vi "gauss.vi"() -> ()   [LabVIEW 2018]
uses:
  Control 1.ctl
  <vilib>/Analysis/4window.llb/windowTd.ctl
  <vilib>/DAQmx/write.llb/DAQmx Write (Analog 1D Wfm NChan NSamp).vi
  <vilib>/Analysis/1siggen.llb/General Gauss-Mod Sine.vi
  <vilib>/measure/maspectr.llb/FFT Power Spectrum and PSD for 1 Chan.vi
  <vilib>/DAQmx/create/channels.llb/DAQmx Create Channel (AO-Voltage-Basic).vi
  <vilib>/DAQmx/configure/timing.llb/DAQmx Timing (Sample Clock).vi
  <vilib>/DAQmx/miscellaneous.llb/DAQmx Fill In Error Info.vi
  <vilib>/Analysis/NI_AALBase.lvlib
  <vilib>/measure/NI_MAPro.lvlib
  <resource>/objmgr/daqmx.rc
  <vilib>/measure/NI_MABase.lvlib
  <vilib>/Analysis/NI_AALPro.lvlib
panel:
  in  "amplitude":dbl=1.0
  in  "delay":dbl
  in  "width":dbl=0.5
  out "Sampling rate":dbl=799999.9999999999
  in  "f2":dbl=300.0 format="%0.2f"
  in  "f1":dbl=100.0 format="%0.2f"
  in  "Test device":bool
  in  "Exit":bool
  out "Actual Sample Rate 2":dbl=800000.0 format="%0.2f"
  in  "Physical Channel(s)":tag="Dev3/ao0:1"
  in  "Min Voltage 2":dbl=-10.0
  in  "Max Voltage 2":dbl=10.0
  in  "Sample Clock Source":tag="OnboardClock"
  in  "Sample Rate 2":dbl=800000.0 format="%#_6p"
  in  "Pulser Cycles":i32=10
  out "Sample per Channel AO":dbl=26666.0
  in  "Pulse generator":T2={"Waveform Type"=2, "Amplitude"=1.0, "Frequency"=300.0} {"Frequency" format="%0.2p"; "Amplitude" format="%0.2p"; "Waveform Type" items=["Sine Wave", "Triangle Wave", "Square Wave", "Sawtooth Wave"]}
  in  "Duty cycle %":dbl=50.0 format="%#.2f"
  in  "samples 2":i32=300
  in  "Amplitude & Delay":cluster{"Amplitude":dbl, "Delay (s)":dbl}[](array[cluster])=[{"Amplitude"=5.0, "Delay (s)"=1.0}, {"Amplitude"=3.0, "Delay (s)"=8.0}, {"Amplitude"=1.0, "Delay (s)"=15.0}]
  in  "interpolation method":i32(ring)=1 items=["nearest", "linear", "spline", "cubic Hermite"]
  out "Pulse Train":waveform(dbl)(graph)={"t0"=timestamp(0 s since 1904-01-01), "dt"=1.25e-06, "Y"=[]}
  out "Waveform Graph 2":cluster{"f0":dbl, "df":dbl, "magnitude":dbl[]}[](graph)=[{"f0"=0.0, "df"=20.0, "magnitude"=array[20000 elements]}, {"f0"=0.0, "df"=20.0, "magnitude"=array[20000 elements]}, {"f0"=0.0, "df"=20.0, "magnitude"=array[20000 elements]}]
  in  "normalized bandwidth":dbl=0.5
  in  "attenuation (dB)":dbl=7.0
  out "Waveform Graph":waveform(dbl)[](graph)=[{"t0"=timestamp(0 s since 1904-01-01), "dt"=1.25e-06, "Y"=array[40000 elements]}, {"t0"=timestamp(0 s since 1904-01-01), "dt"=1.25e-06, "Y"=array[40000 elements]}, {"t0"=timestamp(0 s since 1904-01-01), "dt"=1.25e-06, "Y"=array[40000 elements]}]
  in  "center frequency (Hz)":dbl=200.0
  in  "delay (s)":dbl=0.025
  in  "delta t (s)":dbl=1.25e-06
  in  "samples":i32=40000
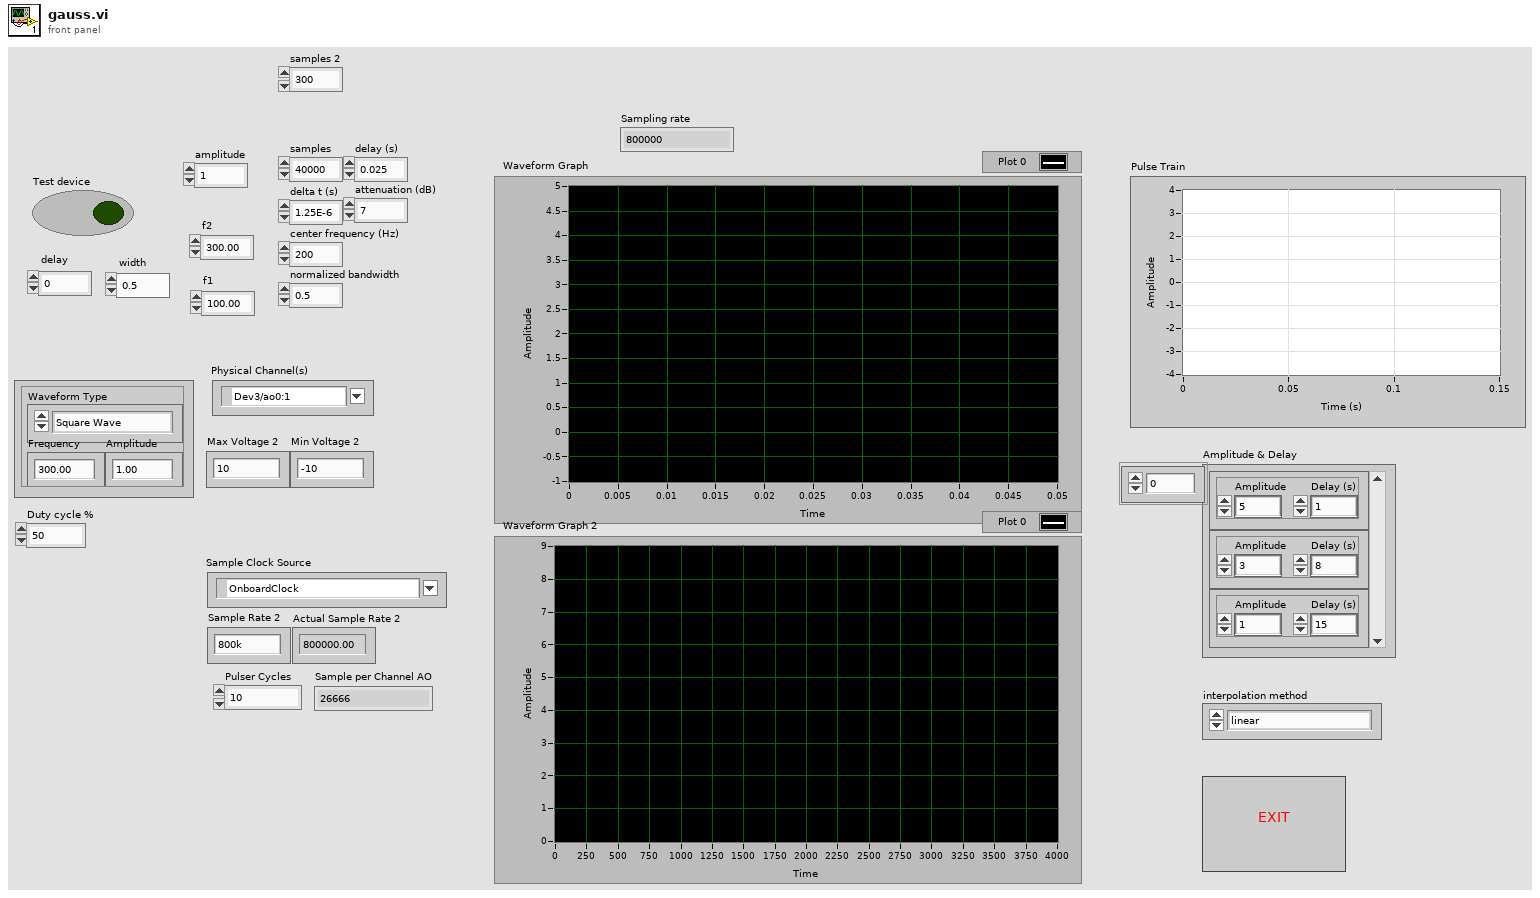
[diagram p1: front panel]
types:
  T1 = typedef "Control 1.ctl" = dbl
  T2 = cluster{"Waveform Type":u16, "Amplitude":T1, "Frequency":dbl}
  T3 = typedef "NI_AALPro.lvlib/windowTd.ctl" = u32
  T4 = enum16{"Sine Wave", "Triangle Wave", "Square Wave", "Sawtooth Wave"}
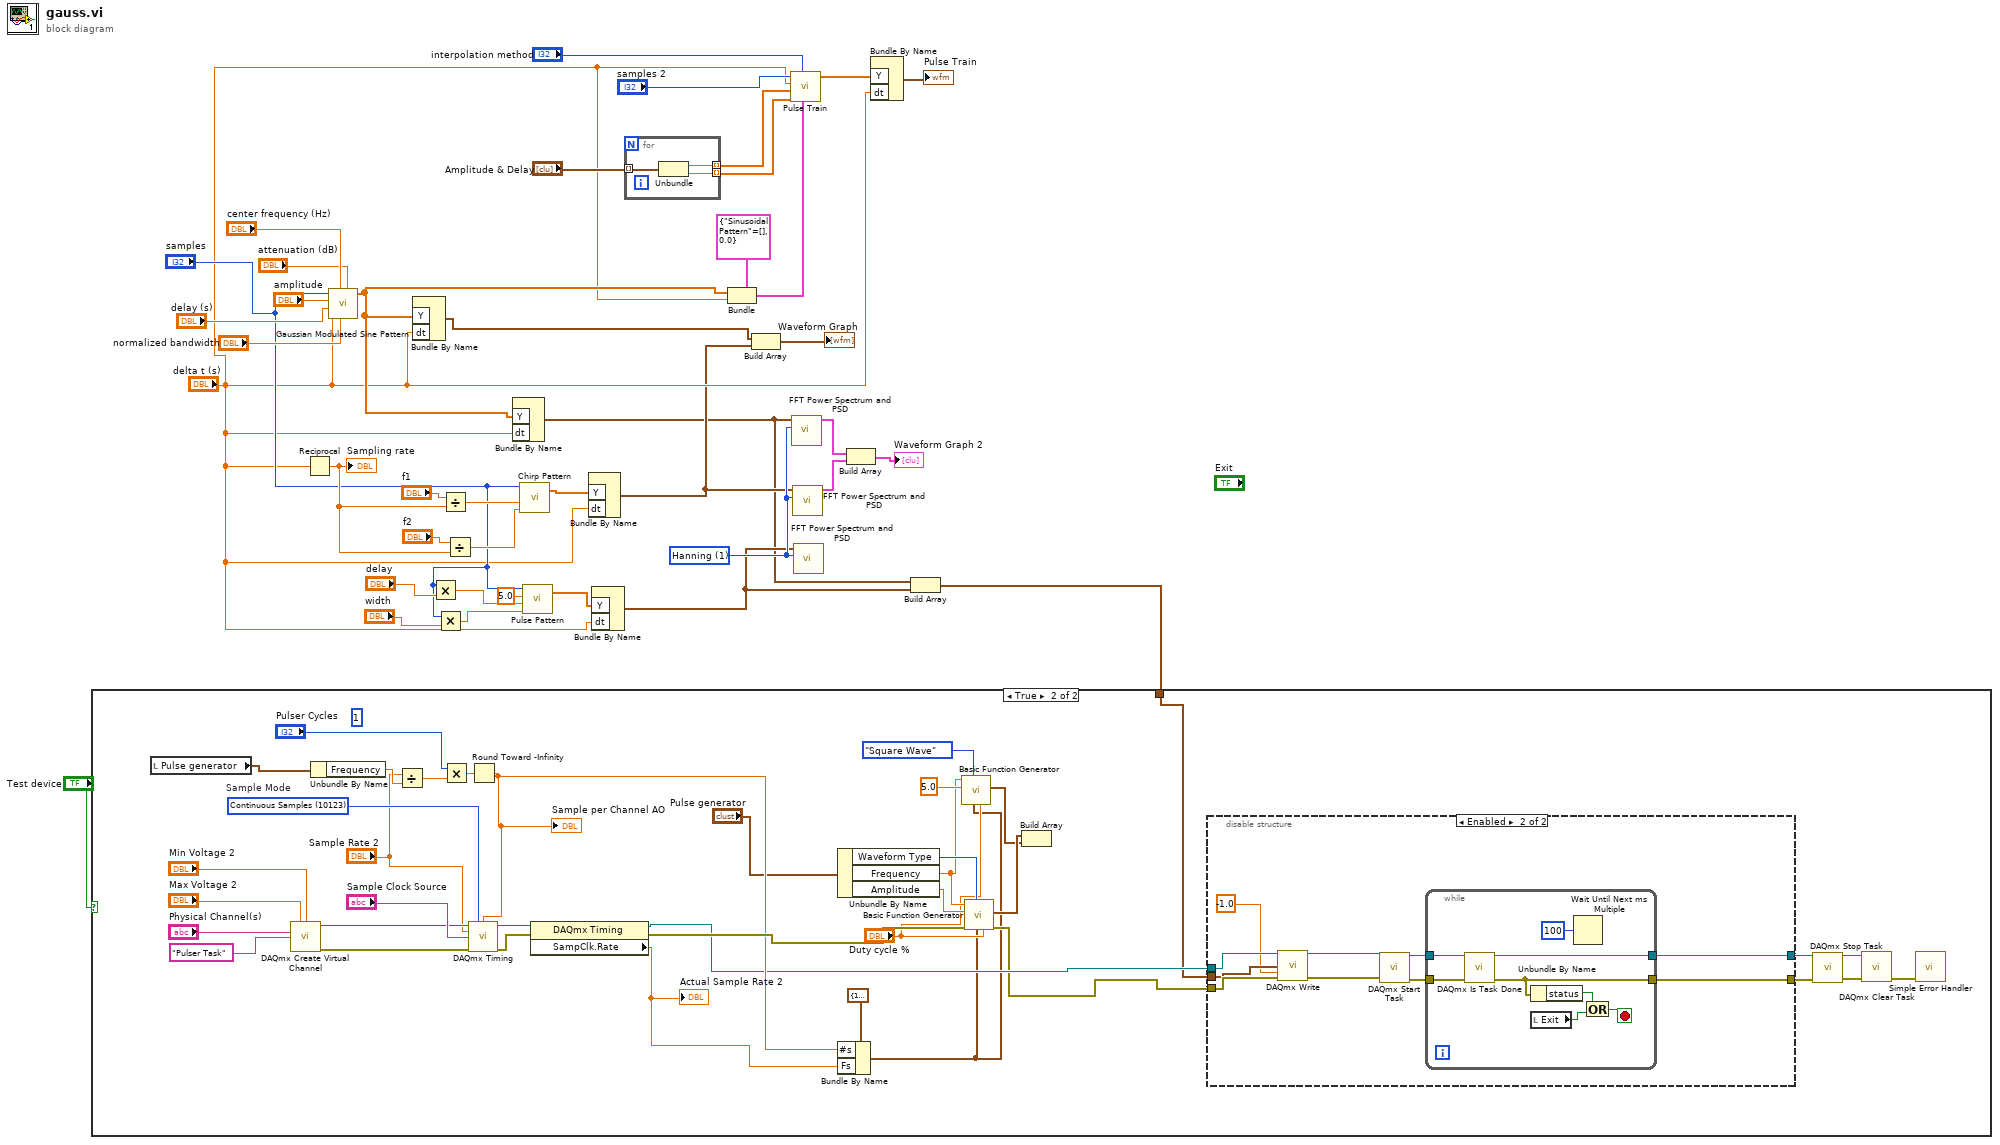
[diagram p0: block diagram]
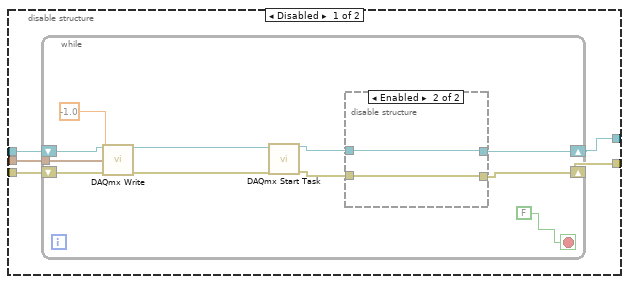
[diagram p3: hidden frame]
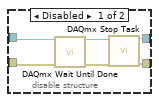
[diagram p4: hidden frame]
diagram:
  w8 = T3 1 items=["Rectangle"=0, "Hanning"=1, "Hamming"=2, "Blackman-Harris"=3, "Exact Blackman"=4, "Blackman"=5, "Flat Top"=6, "4 Term B-Harris "=7, "7 Term B-Harris"=8, "Low Sidelobe"=9, "Blackman Nuttall"=11, "Triangle"=30, "Bartlett-Hanning"=31, "Bohman"=32, "Parzen"=33, "Welch"=34, "Kaiser"=60, "Dolph-Chebyshev"=61, "Gaussian"=62] ("window")
  n1 = Reciprocal(x="delta t (s)") -> (1/x=w14:dbl)
  "Sampling rate" <- w14
  n2 = call <vilib>:"Gaussian Modulated Sine Pattern.vi"("attenuation (dB)"="attenuation (dB)", "normalized bandwidth"="normalized bandwidth", "center frequency (Hz)"="center frequency (Hz)", "delta t (s)"="delta t (s)", "delay (s)"="delay (s)", "amplitude"="amplitude", "samples"="samples") -> ("Gauss-Mod Sine Pattern"=w28:dbl[])  [unwired: 3 in, 1 out]
  n3 = Bundle By Name("Y"=w28, "dt"="delta t (s)") -> (w25:waveform(dbl))  [unwired: 1 in]
  n4 = Multiply(x="samples", y="delay") -> (x*y=w9:dbl)
  n5 = Multiply(x="samples", y="width") -> (x*y=w10:dbl)
  n6 = Divide(x="f1", y=w14) -> (x/y=w21:dbl)
  n7 = Divide(x="f2", y=w14) -> (x/y=w19:dbl)
  n8 = Bundle By Name("Y"=w28, "dt"="delta t (s)") -> (w1:waveform(dbl))  [unwired: 1 in]
  n9 = call <vilib>:"Chirp Pattern.vi"("f2"=w19, "f1"=w21, "samples"="samples") -> ("Chirp Pattern"=w23:dbl[])  [unwired: 1 in, 1 out]
  n10 = call <vilib>:"Pulse Pattern.vi"("width"=w10, "delay"=w9, "amplitude"=5.0, "samples"="samples") -> ("Pulse Pattern"=w15:dbl[])  [unwired: 1 out]
  n11 = Bundle By Name("Y"=w23, "dt"="delta t (s)") -> (w2:waveform(dbl))  [unwired: 1 in]
  n12 = Bundle By Name("Y"=w15, "dt"="delta t (s)") -> (w6:waveform(dbl))  [unwired: 1 in]
  n13 = for {
    tunnel: "Amplitude & Delay" -> [w43] mode=indexing
    tunnel: [w42] -> w32 mode=indexing
    tunnel: [w41] -> w31 mode=indexing
    n14 = Unbundle(w43) -> ("Amplitude"=w42:dbl, "Delay (s)"=w41:dbl)
  }
  n15 = Bundle(cluster=cluster{"Sinusoidal Pattern":dbl[], dbl} {"Sinusoidal Pattern"=[], 0.0} ("output cluster"), "Sinusoidal Pattern"=w28, "delta t (s)") -> (w27:cluster{"Sinusoidal Pattern":dbl[], dbl})
  n16 = Build Array(w25, w2) -> (→"Waveform Graph":waveform(dbl)[])
  n17 = call <vilib>:"Pulse Train.vi"("prototype spec"=w27, "interpolation method"="interpolation method", "Delay (s)"=w31, "Amplitude"=w32, "delta t of pulse train (s)"="delta t (s)", "samples"="samples 2") -> ("Pulse Train"=w35:dbl[])  [unwired: 4 in, 1 out]
  n18 = call-poly <vilib>:"FFT Power Spectrum and PSD.vi"("window"=w8, "time signal"=w1) -> ("Power Spectrum / PSD"=w17:cluster{"f0":dbl, "df":dbl, "magnitude":dbl[]})  [unwired: 6 in, 3 out]
  n19 = call-poly <vilib>:"FFT Power Spectrum and PSD.vi"("window"=w8, "time signal"=w2) -> ("Power Spectrum / PSD"=w18:cluster{"f0":dbl, "df":dbl, "magnitude":dbl[]})  [unwired: 6 in, 3 out]
  n20 = call-poly <vilib>:"FFT Power Spectrum and PSD.vi"("window"=w8, "time signal"=w6) -> ()  [unwired: 6 in, 4 out]
  n21 = Build Array(w17, w18) -> (→"Waveform Graph 2":cluster{"f0":dbl, "df":dbl, "magnitude":dbl[]}[])
  n22 = Bundle By Name("Y"=w35, "dt"="delta t (s)") -> (→"Pulse Train":waveform(dbl))  [unwired: 1 in]
  n23 = Build Array(w1, w6) -> (w5:waveform(dbl)[])
  n24 = case shown="True" "Test device" {
    tunnel: w5 -> [_ w44]
    frame False {
    }
    frame True {
      (unwired) 1 ("x")
      w79 = 10123 items=["Finite Samples"=10178, "Continuous Samples"=10123, "Hardware Timed Single Point"=12522]  # Sample Mode
      n25 = local read "Pulse generator"() -> (w63:T2)
      n26 = call-poly <vilib>:"DAQmx Create Virtual Channel.vi"("maximum value"="Max Voltage 2", "minimum value"="Min Voltage 2", "physical channels"="Physical Channel(s)", "name to assign"="Pulser Task") -> ("task out"=w70:refnum<k21>, "error out"=w69:errorcluster)  [unwired: 10 in]
      n27 = Unbundle By Name(w63) -> ("Frequency"=w68:dbl)
      n28 = Divide(x="Sample Rate 2", y=w68) -> (x/y=w66:dbl)
      n29 = Multiply(x="Pulser Cycles", y=w66) -> (x*y=w65:dbl)
      n30 = Round Toward -Infinity(1:w65) -> (0:w64:dbl)
      "Sample per Channel AO" <- w64
      n31 = call-poly <vilib>:"DAQmx Timing.vi"("task/channels in"=w70, "sample mode"=w79, "samples per channel"=w64, "rate"="Sample Rate 2", "source"="Sample Clock Source", "error in"=w69) -> ("task out"=w81:refnum<k21>, "error out"=w80:errorcluster)  [unwired: 8 in]
      n32 = property class="DAQmx Timing"(reference=w81, error in=w80) -> (reference out=w62:refnum<k21>, error out=w73:errorcluster, "SampClk.Rate"=w71:dbl)
      "Actual Sample Rate 2" <- w71
      n33 = Unbundle By Name("Pulse generator") -> ("Waveform Type"=w60:u16, "Frequency"=w56:dbl, "Amplitude"=w59:T1)
      n34 = Bundle By Name(cluster=cluster{"Fs":dbl, "#s":dbl} {"Fs"=1000.0, "#s"=1000.0} ("sampling info"), "#s"=w64, "Fs"=w71) -> (w51:cluster{"Fs":dbl, "#s":dbl})
      n35 = call <vilib>:"Basic Function Generator.vi"("square wave duty cycle (%)"="Duty cycle %", "sampling info"=w51, "signal type"=T4."Square Wave", "amplitude"=5.0, "frequency"=w56) -> ("signal out"=w52:waveform(dbl))  [unwired: 4 in, 2 out]
      n36 = call <vilib>:"Basic Function Generator.vi"("square wave duty cycle (%)"="Duty cycle %", "sampling info"=w51, "signal type"=w60, "error in (no error)"=w73, "amplitude"=w59, "frequency"=w56) -> ("error out"=w61:errorcluster, "signal out"=w53:waveform(dbl))  [unwired: 3 in, 1 out]
      n37 = Build Array(w53, w52) -> ()  [unwired: 1 out]
      n38 = disable-structure shown="Enabled" {
        disable-tunnel: w44 -> [w86 w109]
        disable-tunnel: [w85 w108] -> w48
        disable-tunnel: [w84 w107] -> w45
        disable-tunnel: w62 -> [w83 w111]
        disable-tunnel: w61 -> [w82 w110]
        frame Disabled {
          n39 = while {
            tunnel: w86 -> [w97]
            shift-right: [w93] -> w85
            shift-left: w83 -> [w91]
            shift-right: [w92] -> w84
            shift-left: w82 -> [w90]
            stop <- FALSE stop-if-true
            n40 = call-poly <vilib>:"DAQmx Write.vi"("task/channels in"=w91, "data"=w97, "timeout"=-1.0, "error in"=w90) -> ("task out"=w96:refnum<k21>, "error out"=w95:errorcluster)  [unwired: 9 in, 1 out]
            n41 = call <vilib>:"DAQmx Start Task.vi"("task/channels in"=w96, "error in"=w95) -> ("task out"=w89:refnum<k21>, "error out"=w88:errorcluster)  [unwired: 12 in]
            n42 = disable-structure shown="Enabled" {
              disable-tunnel: [w103 w105] -> w93
              disable-tunnel: [w102 w104] -> w92
              disable-tunnel: w89 -> [w101 w105]
              disable-tunnel: w88 -> [w100 w104]
              frame Disabled {
                n43 = call <vilib>:"DAQmx Wait Until Done.vi"("task/channels in"=w101, "error in"=w100) -> ("task out"=w99:refnum<k21>, "error out"=w98:errorcluster)  [unwired: 12 in]
                n44 = call <vilib>:"DAQmx Stop Task.vi"("task/channels in"=w99, "error in"=w98) -> ("task out"=w103:refnum<k21>, "error out"=w102:errorcluster)  [unwired: 12 in]
              }
              frame Enabled {
              }
            }
          }
        }
        frame Enabled {
          n45 = call-poly <vilib>:"DAQmx Write.vi"("task/channels in"=w111, "data"=w109, "timeout"=-1.0, "error in"=w110) -> ("task out"=w113:refnum<k21>, "error out"=w115:errorcluster)  [unwired: 9 in, 1 out]
          n46 = call <vilib>:"DAQmx Start Task.vi"("task/channels in"=w113, "error in"=w115) -> ("task out"=w112:refnum<k21>, "error out"=w114:errorcluster)  [unwired: 12 in]
          n47 = while {
            tunnel: w112 -> [w123]
            tunnel: w114 -> [w122]
            tunnel: [w120] -> w107
            tunnel: [w121] -> w108
            stop <- w117 stop-if-true
            n48 = call <vilib>:"DAQmx Is Task Done.vi"("task/channels in"=w123, "error in"=w122) -> ("task out"=w121:refnum<k21>, "error out"=w120:errorcluster)  [unwired: 11 in, 1 out]
            n49 = Unbundle By Name(w120) -> ("status"=w118:bool)
            n50 = local read "Exit"() -> (w116:bool)
            n51 = Wait Until Next ms Multiple(millisecond multiple=u32 100) -> ()  [unwired: 1 out]
            n52 = Compound Arithmetic op=OR(w118, w116) -> (w117:bool)
          }
        }
      }
      n53 = call <vilib>:"DAQmx Stop Task.vi"("task/channels in"=w48, "error in"=w45) -> ("task out"=w47:refnum<k21>, "error out"=w46:errorcluster)  [unwired: 12 in]
      n54 = call <vilib>:"DAQmx Clear Task.vi"("task in"=w47, "error in"=w46) -> ("error out"=w78:errorcluster)  [unwired: 13 in]
      n55 = call <vilib>:"Simple Error Handler.vi"("error in (no error)"=w78) -> ()  [unwired: 4 in, 5 out]
    }
  }
